vi "X_Phik.vi"(3 "Lq":i32, 4 "u":dbl format="%#_13g") -> (1 "phik":dbl[](array[numeric]))   [LabVIEW 2019]
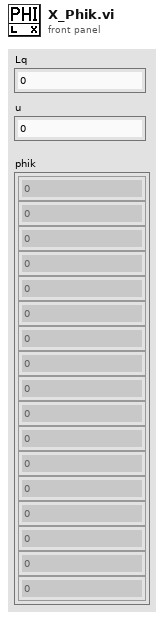
[diagram p1: front panel]
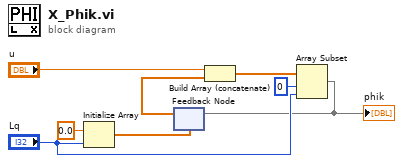
[diagram p0: block diagram]
diagram:
  n1 = Initialize Array(0.0 ("element"), "Lq") -> (w7:dbl[])
  n2 = feedback #1(w7) -> (w8:dbl[])
  n3 = Build Array (concatenate)("u", w8) -> (w4:dbl[])
  n4 = Array Subset(array=w4, index=0, length="Lq") -> (w1:dbl[])
  "phik" <- w1
  n5 = feedback-in #1(w1) -> ()
